vi "Get Node by Address.vi"(8 "error in":errorcluster, 10 "Address":i32[](array[numeric]), 11 "XML Document in":refnum<class "XML Document.lvclass">) -> (0 "error out":errorcluster, 1 "Found?":bool, 2 "Node.lvclass":refnum<class "Node.lvclass">, 3 "XML Document out":refnum<class "XML Document.lvclass">)   [LabVIEW 2014, in "XML Document.lvclass"]
uses:
  XML Document.lvclass
  Node_class/Node.lvclass
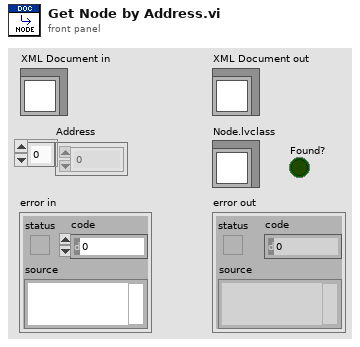
[diagram p1: front panel]
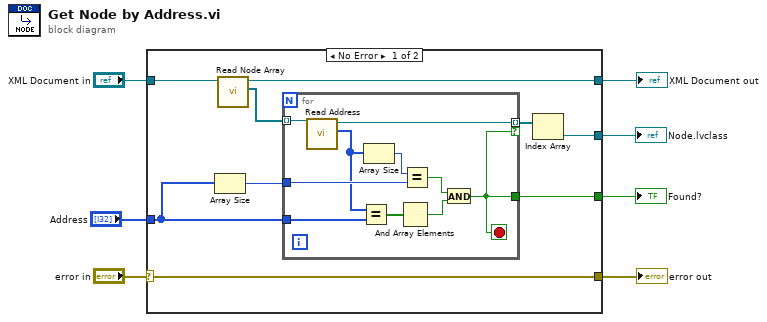
[diagram p0: block diagram]
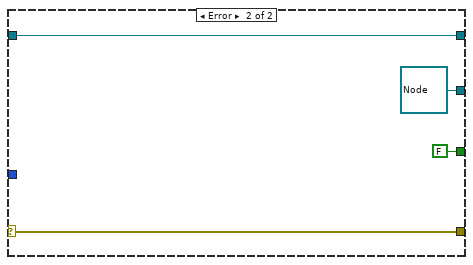
[diagram p2: hidden frame]
diagram:
  n1 = case shown="No Error" "error in" {
    selector: "error in" -> [w15 w30]
    tunnel: [w15 w30] -> w6
    tunnel: [w14 w29] -> w4
    tunnel: "XML Document in" -> [w16 w29]
    tunnel: "Address" -> [w11 _]
    tunnel: [w9 refnum<class "Node.lvclass"> refnum ("Node.lvclass")] -> w2
    tunnel: [w8 FALSE] -> w1
    frame No Error {
      n2 = Array Size(array=w11) -> (size(s)=w12:i32)
      n3 = call-dynamic "Read Node Array.vi"("XML Document in"=w16) -> ("Node Array"=w13:refnum<class "Node.lvclass">[], "XML Document out"=w14:refnum<class "XML Document.lvclass">)  [unwired: 8 in, 1 out]
      n4 = for {
        tunnel: w13 -> [w19] mode=indexing
        tunnel: w12 -> [w25]
        tunnel: w11 -> [w23]
        tunnel: [w18] -> w10 mode=indexing if=w17
        tunnel: [w17] -> w8
        stop <- w17 stop-if-true
        n5 = call-dynamic "Read Address.vi"("Node in"=w19) -> ("Address"=w24:i32[], "Node out"=w18:refnum<class "Node.lvclass">)  [unwired: 8 in, 1 out]
        n6 = Equal?(x=w24, y=w23) -> (x = y?=w21:bool[])
        n7 = Array Size(array=w24) -> (size(s)=w26:i32)
        n8 = And Array Elements(Boolean array=w21) -> (logical AND=w20:bool)
        n9 = Equal?(x=w26, y=w25) -> (x = y?=w22:bool)
        n10 = And(x=w22, y=w20) -> (x .and. y?=w17:bool)
      }
      n11 = Index Array(array=w10) -> (element=w9:refnum<class "Node.lvclass">)  [unwired: 1 in]
    }
    frame Error {
    }
  }
  "error out" <- w6
  "XML Document out" <- w4
  "Node.lvclass" <- w2
  "Found?" <- w1
